vi "ScriptCreateIOselector.vi"(4 "numeric representation":T1=enum."Word", 6 "digital(F)/numeric(T)":bool, 7 "indicator (F)/control (T)":bool, 8 "error in (no error)":errorcluster, 9 "IO names":string[](array[string]), 10 "VI path":path, 11 "Application in":refnum<vi>) -> ()   [LabVIEW 2023]
uses:
  <vilib>/numeric/LVNumericRepresentation.ctl
  <vilib>/eio/EIO_TerminalDirection.ctl
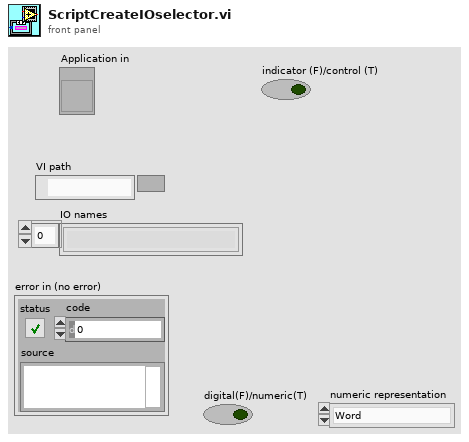
[diagram p1: front panel]
types:
  T1 = typedef "LVNumericRepresentation.ctl" = enum32{"Extended Precision", "Double Precision", "Single Precision", "Long", "Word", "Byte", "Unsigned Long", "Unsigned Word", "Unsigned Byte", "Complex Extended", "Complex Double", "Complex Single", "Quad", "Unsigned Quad", "Fixed-Point"}
  T2 = typedef "EIO_TerminalDirection.ctl" = enum16{"read", "write", "none", "both"}
  T3 = typedef "LVPositionTypeDef.ctl" = cluster{"Left":i32, "Top":i32}
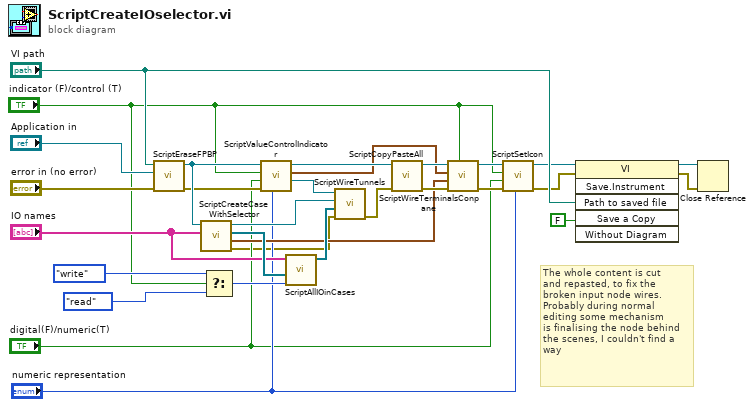
[diagram p0: block diagram]
diagram:
  # "The whole content is cut\nand repasted, to fix the\nbroken input node wires.\nProbably during normal\nediting some mechanism\nis finalising the node behind\nthe scenes, I couldn't find a\nway"
  n1 = call "ScriptEraseFPBP.vi"("error in (no error)"="error in (no error)", "application reference (local)"="Application in", "VI path"="VI path") -> ("error out"=w21:errorcluster, "VI out"=w28:refnum<vi>)  [unwired: 7 in]
  n2 = call "ScriptCreateCaseWithSelector.vi"("I/O names"="IO names", "VI in"=w28) -> ("error out"=w1:errorcluster, "Enum position"=w12:T3, "Case diagrams"=w25:refnum<vi>[], "CaseStructure out"=w26:refnum<vi>)  [unwired: 6 in]
  n3 = Select(t=EIO_TerminalDirection."write" ("direction"), s="indicator (F)/control (T)", f=EIO_TerminalDirection."read" ("direction")) -> (s? t:f=w18:T2)
  n4 = call "ScriptValueControlIndicator.vi"("numeric representation"="numeric representation", "error in (no error)"=w21, "digital(F)/numeric(T)"="digital(F)/numeric(T)", "indicator (F)/control (T)"="indicator (F)/control (T)", "VI in"=w28) -> ("Value terminal"=w15:refnum<vi>, "Value position"=w11:T3, "VI out"=w17:refnum<vi>)  [unwired: 3 in, 1 out]
  n5 = call "ScriptAllIOinCases.vi"("direction"=w18, "Case diagrams"=w25, "I/O names"="IO names") -> ("IO terminals"=w27:refnum<vi>[])  [unwired: 8 in]
  n6 = call "ScriptWireTunnels.vi"("error in"=w1, "i/o terminals"=w27, "CaseStructure in"=w26, "ControlTerminal in"=w15) -> ("error out"=w16:errorcluster)  [unwired: 7 in]
  n7 = call "ScriptCopyPasteAll.vi"("error in (no error)"=w16, "VI in"=w17) -> ("error out"=w14:errorcluster, "VI out"=w13:refnum<vi>)  [unwired: 8 in]
  n8 = call "ScriptWireTerminalsConpane.vi"("indicator (F)/control (T)"="indicator (F)/control (T)", "error in (no error)"=w14, "Enum position"=w12, "Value position"=w11, "VI in"=w13) -> ("error out"=w6:errorcluster, "VI out"=w8:refnum<vi>)  [unwired: 5 in]
  n9 = call "ScriptSetIcon.vi"("numeric representation"="numeric representation", "error in (no error)"=w6, "digital(F)/numeric(T)"="digital(F)/numeric(T)", "indicator (F)/control (T)"="indicator (F)/control (T)", "VI reference"=w8) -> ("error out"=w5:errorcluster, "VI reference out"=w7:refnum<vi>)  [unwired: 5 in]
  n10 = invoke class="VI" method="Save.Instrument"(reference=w7, error in=w5, "Path to saved file"="VI path", "Save a Copy"=FALSE) -> (reference out=w22:refnum<vi>, error out=w23:errorcluster)  [unwired: 2 in, 4 out]
  n11 = Close Reference(reference=w22, error in (no error)=w23) -> ()  [unwired: 1 out]
